vi "Pipelined Burst FFT Core FXP (BlockFloat).vi"(9 "xn_im":fxp<+/-,20,2>, 10 "xn_re":fxp<+/-,20,2>, 11 "FFT State Info In":T2) -> (0 "Output Valid":bool, 1 "Block Exponent":fxp<+,5,5>, 2 "FFT Output":T1, 4 "xk_index":fxp<+,11,11>, 6 "Done":bool)   [LabVIEW 2011]
uses:
  <vilib>/rvi/IPIntegrationNode/IPINode_Utilities/niFpgaIPINodeSimCore.vi
  <vilib>/rvi/FXPMathLib/basic elements/FxpDiscreteDelay/XNode/nifxpmath_DiscreteDelay.xnode
  <vilib>/rvi/XilinxIP/XIPIN_XNode/niFpgaXIPIN.xnode
  <userlib>/FPGA Library/Code Development/Signal Processing/FFT/Pipelined Burst FFT/Xilinx FFT Core Block Float/BlockFloatFFT_E46F351946EF808103B13FA465BCBB50.dll
  <vilib>/rvi/IPIntegrationNode/IPINode_Xnode/niFpgaIPINode.xnode
panel:
  out "xk_re":fxp<+/-,20,2>
  out "xk_im":fxp<+/-,20,2>
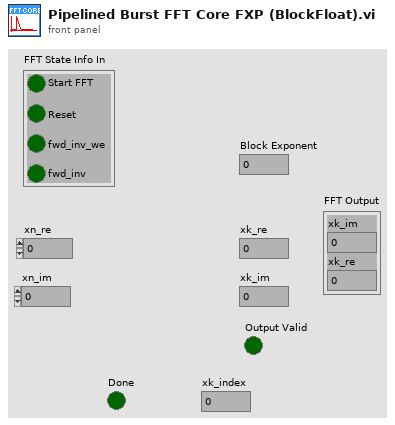
[diagram p1: front panel]
types:
  T1 = cluster{"xk_im":fxp<+/-,20,2>, "xk_re":fxp<+/-,20,2>}
  T2 = cluster{"Reset":bool, "Start FFT":bool, "fwd_inv_we":bool, "fwd_inv":bool}
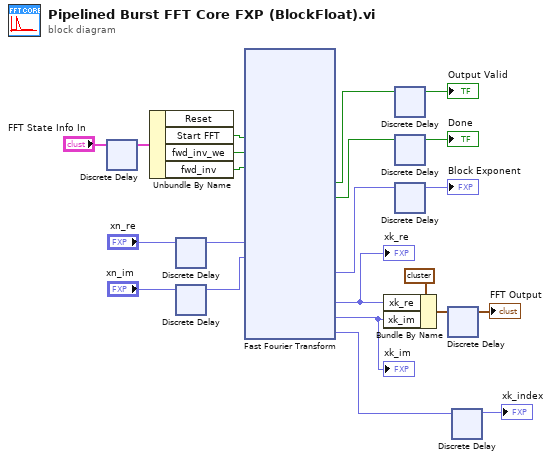
[diagram p0: block diagram]
diagram:
  n1 = xnode "Discrete Delay"("D"="FFT State Info In") -> ("Q"=w18:T2)
  n2 = Unbundle By Name(w18) -> ("Start FFT"=w15:bool, "fwd_inv_we"=w14:bool, "fwd_inv"=w13:bool)  [unwired: 1 out]
  n3 = xnode "Discrete Delay"("D"="xn_re") -> ("Q"=w12:fxp<+/-,20,2>)
  n4 = xnode "Discrete Delay"("D"="xn_im") -> ("Q"=w11:fxp<+/-,20,2>)
  n5 = xnode ("Fast Fourier Transform")("start"=w15, "fwd_inv"=w14, "fwd_inv_we"=w13, "xn_re"=w12, "xn_im"=w11) -> ("dv"=w7:bool, "done"=w4:bool, "blk_exp"=w6:fxp<+,5,5>, "xk_re"=w9:fxp<+/-,20,2>, "xk_im"=w8:fxp<+/-,20,2>, "xk_index"=w1:fxp<+,11,11>)  [unwired: 4 out]
  "xk_im" <- w8
  "xk_re" <- w9
  n6 = Bundle By Name(cluster=T1 {"xk_im"=0.0, "xk_re"=0.0} ("FFT Output"), "xk_re"=w9, "xk_im"=w8) -> (w19:T1)
  n7 = xnode "Discrete Delay"("D"=w7) -> ("Q"=→"Output Valid":bool)
  n8 = xnode "Discrete Delay"("D"=w4) -> ("Q"=→"Done":bool)
  n9 = xnode "Discrete Delay"("D"=w6) -> ("Q"=→"Block Exponent":fxp<+,5,5>)
  n10 = xnode "Discrete Delay"("D"=w19) -> ("Q"=→"FFT Output":T1)
  n11 = xnode "Discrete Delay"("D"=w1) -> ("Q"=→"xk_index":fxp<+,11,11>)
